vi "Email Shifter about Out-of-range Devices.vi"(8 "error in":errorcluster, 10 "Recipients":string[](array[string])=["plane1@hawk.iit.edu"], 11 "Summary Listbox":refnum<vi>) -> (0 "error out":errorcluster)   [LabVIEW 2013, in "ACNET Monitor.lvlib"]
uses:
  ACNET Monitor.lvlib
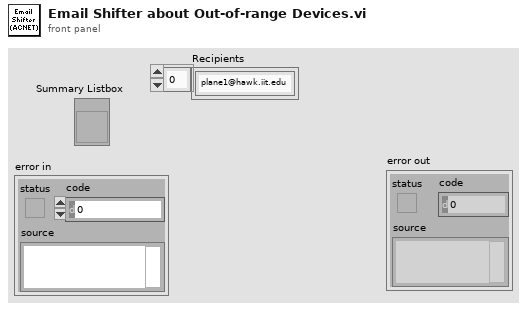
[diagram p1: front panel]
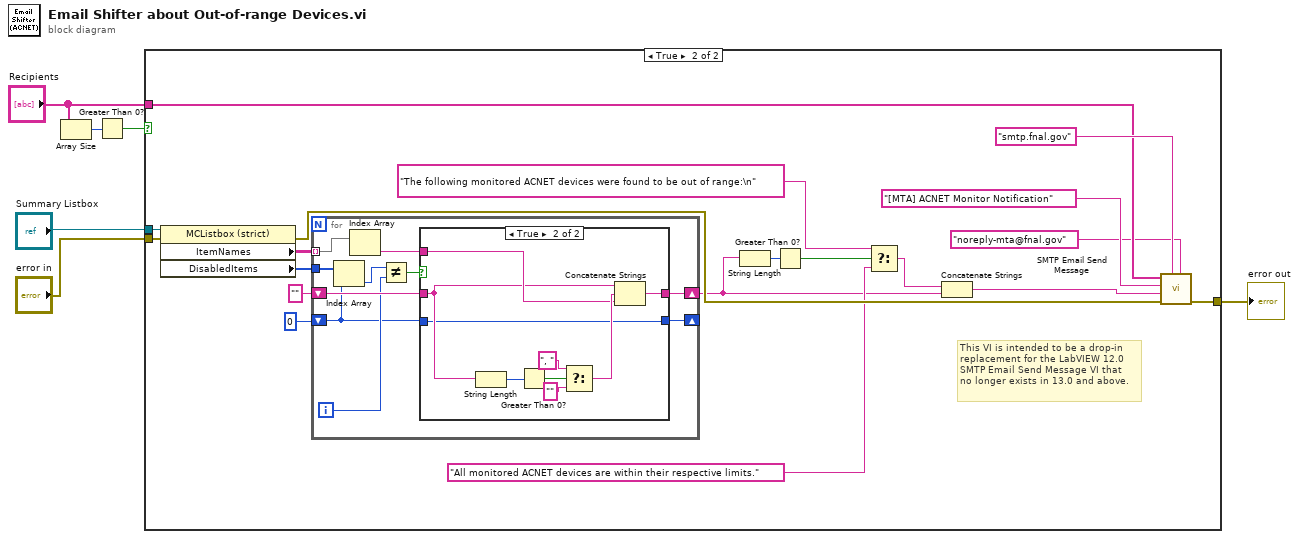
[diagram p0: block diagram]
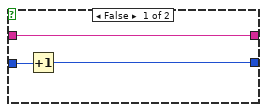
[diagram p3: hidden frame]
diagram:
  n1 = Array Size(array="Recipients") -> (size(s)=w2:i32)
  n2 = Greater Than 0?(x=w2) -> (x > 0?=w1:bool)
  n3 = case shown="True" w1 {
    tunnel: "Summary Listbox" -> [_ w26]
    tunnel: "error in" -> [w7 w25]
    tunnel: [w7 w23] -> w4
    tunnel: "Recipients" -> [_ w9]
    frame False {
    }
    frame True {
      # "This VI is intended to be a drop-in\nreplacement for the LabVIEW 12.0\nSMTP Email Send Message VI that\nno longer exists in 13.0 and above."
      n4 = property class="MCListbox (strict)"(reference=w26, error in=w25) -> (error out=w24:errorcluster, "ItemNames"=w19:string[][], "DisabledItems"=w18:i32[])  [unwired: 1 out]
      n5 = for {
        tunnel: w19 -> [w28] mode=indexing
        shift-right: [w35] -> w11
        shift-left: "" -> [w36]
        tunnel: w18 -> [w31]
        shift-right: [w32] -> _
        shift-left: u32 0 -> [w30]
        i -> [w34]
        n6 = Index Array(array=w31, index=w30) -> (element=w29:i32)
        n7 = Index Array(array=w28) -> (element=w27:string)  [unwired: 1 in]
        n8 = Not Equal?(x=w29, y=w34) -> (x != y?=w33:bool)
        n9 = case shown="True" w33 {
          tunnel: w36 -> [w37 w42]
          tunnel: [w37 w44] -> w35
          tunnel: w30 -> [w39 w40]
          tunnel: [w38 w40] -> w32
          tunnel: w27 -> [_ w43]
          frame False {
            n10 = Increment(x=w39) -> (x+1=w38:u32)
          }
          frame True {
            n11 = String Length(string=w42) -> (length=w41:i32)
            n12 = Greater Than 0?(x=w41) -> (x > 0?=w48:bool)
            n13 = Select(t=", " ("element"), s=w48, f="" ("element")) -> (s? t:f=w45:string)
            n14 = Concatenate Strings(w42, w45, w43) -> (w44:string)
          }
        }
      }
      n15 = String Length(string=w11) -> (length=w16:i32)
      n16 = Greater Than 0?(x=w16) -> (x > 0?=w15:bool)
      n17 = Select(t="The following monitored ACNET devices were found to be out of range:\n" ("element"), s=w15, f="All monitored ACNET devices are within their respective limits." ("element")) -> (s? t:f=w12:string)
      n18 = Concatenate Strings(w12, w11) -> (w10:string)
      n19 = call "SMTP Email Send Message.vi"("sender"="noreply-mta@fnal.gov", "server"="smtp.fnal.gov", "error in (no error)"=w24, "message"=w10, "subject"="[MTA] ACNET Monitor Notification" ("Subject"), "recipients"=w9) -> ("error out"=w23:errorcluster)  [unwired: 5 in]
    }
  }
  "error out" <- w4
